vi "Write Message Header.vi"(8 "error in (no error)":errorcluster, 10 "Message Header":u8[](array[numeric]), 11 "SECS-II Class in":refnum<class "SECS-II Class.lvclass">) -> (0 "error out":errorcluster, 3 "SECS-II Class out":refnum<class "SECS-II Class.lvclass">)   [LabVIEW 2020, in "SECS Communication.lvlib" / "SECS-II Class.lvclass"]
uses:
  SECS-II Class.lvclass
  SECS-II Class.lvclass/SECS-II Class.ctl
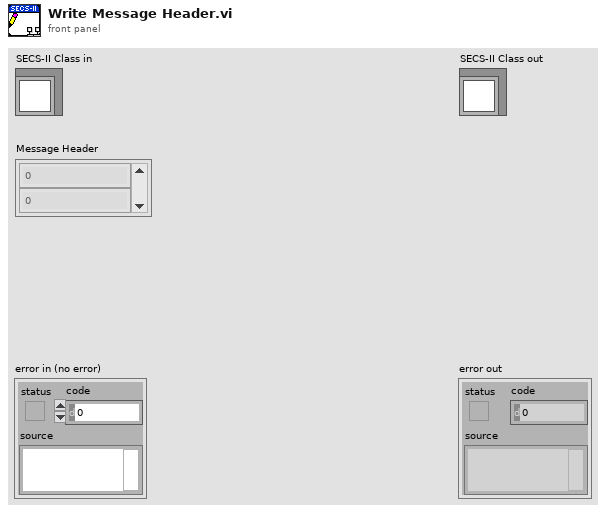
[diagram p1: front panel]
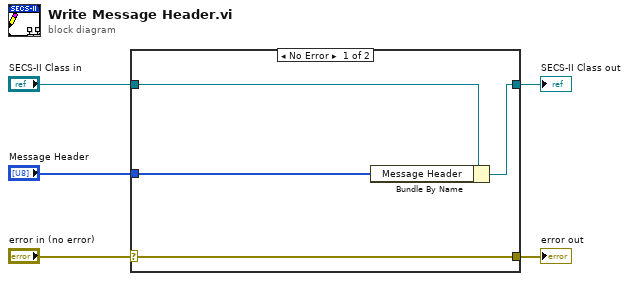
[diagram p0: block diagram]
diagram:
  n1 = case shown="No Error" "error in (no error)" {
    selector: "error in (no error)" -> [w9 w10]
    tunnel: [w9 w10] -> w4
    tunnel: [w7 w11] -> w2
    tunnel: "SECS-II Class in" -> [w8 w11]
    tunnel: "Message Header" -> [w6 _]
    frame No Error {
      n2 = Bundle By Name(cluster=w8, "Message Header"=w6) -> (w7:refnum<class "SECS-II Class.lvclass">)
    }
    frame Error {
    }
  }
  "error out" <- w4
  "SECS-II Class out" <- w2
